vi "Write Top level parent.vi"(8 "error in (no error)":errorcluster, 10 "Top level parent":refnum<vi>, 11 "D_Datagrid in":refnum<class "D_Datagrid.lvclass">) -> (0 "error out":errorcluster, 3 "D_Datagrid out":refnum<class "D_Datagrid.lvclass">)   [LabVIEW 2018, in "D Datagrid Library.lvlib" / "D_Datagrid.lvclass"]
uses:
  D_Datagrid.lvclass
  D_Datagrid.lvclass/D_Datagrid.ctl
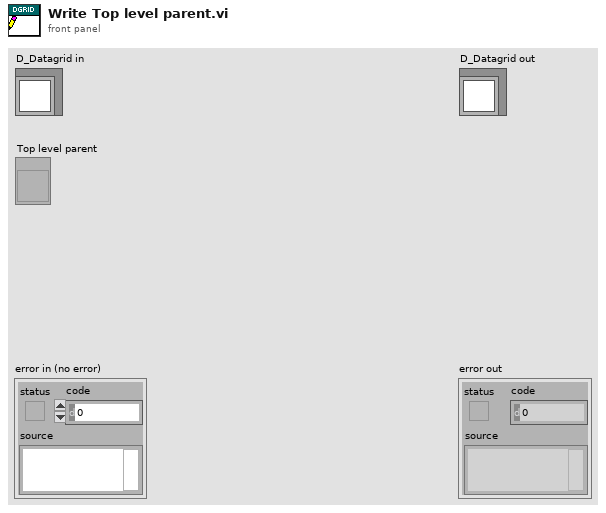
[diagram p1: front panel]
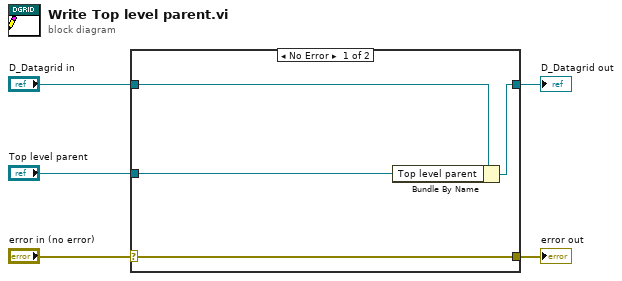
[diagram p0: block diagram]
diagram:
  n1 = case shown="No Error" "error in (no error)" {
    selector: "error in (no error)" -> [w9 w10]
    tunnel: [w9 w10] -> w4
    tunnel: [w7 w11] -> w2
    tunnel: "D_Datagrid in" -> [w8 w11]
    tunnel: "Top level parent" -> [w6 _]
    frame No Error {
      n2 = Bundle By Name(cluster=w8, "Top level parent"=w6) -> (w7:refnum<class "D_Datagrid.lvclass">)
    }
    frame Error {
    }
  }
  "error out" <- w4
  "D_Datagrid out" <- w2
